vi "Main.vi"() -> ()   [LabVIEW 2020, in "Rename to match project.lvlib"]
uses:
  Rename to match project.lvlib
  process loops/Instrument Manager/Instrument State.ctl
  process loops/UI Manager/Data Display Loop Data.ctl
  process loops/Logging/Logging Configuration.ctl
  process loops/UI Manager/UI Data.ctl
  process loops/UI Manager/UI Display State.ctl
  Typedefs/System Control Data.ctl
  <vilib>/Utility/error.llb/Error Cluster From Error Code.vi
  <vilib>/ErrorRing/Error Ring.xnode
  support/Message Queue/Message Queue.lvlib
  support/User Event - Stop/User Event - Stop.lvlib
  process loops/Instrument Manager/Instrument Manager.lvlib
  process loops/Acquisition/Acquisition.lvlib
  process loops/Remote Connection Manager/Remote Connection Manager.lvlib
  process loops/Logging/Logging.lvlib
panel:
  in  "Time Interval (sec)":i32=1200
  out "Data Graph":cluster{timestamp[], dbl[]}[](graph)
  in  "Config Log Btn":bool
  in  "Sampling rate\n(sec/sample)":dbl=1.0 min=0.1 step=0.1
  in  "Log Data":bool
  in  "Stop Btn":bool=TRUE
  in  "Run Btn":bool
  out "Data Ind":dbl format="%d <u>"
  in  "Setpoint (units)":dbl format="%.3f"
  out "VISA resource":refnum<visa-resource-name>
  # "Plugin Template"
  # "Config"
  # "#CodeRecommended - To change display units, or remove them entirely, right click the display indicator >> Properties >> Display Format and replace or delete the <u>. If the rest of the format string is changed, be sure to change the Display Units cases in the UI Manager loop on the Block Diagram to reflect the changes."
  # "#CodePossibility - When plotting additional Instrument State data, right-click the Data Graph >> Properties >> Appearance and change the number of plots shown. Then go to the Plots tab and rename the plots to reflect the data being displayed."
  # "Instrument Control"
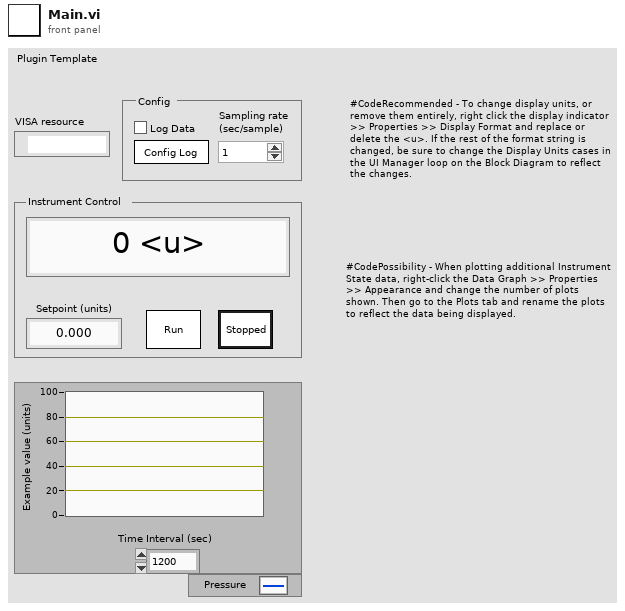
[diagram p1: front panel]
types:
  T1 = typedef "Rename to match project.lvlib/Data Display Loop Data.ctl" = cluster{"Data Timestamps":timestamp[], "Data Values":dbl[], "Previous Run State":bool}
  T2 = typedef "Rename to match project.lvlib/Instrument Manager.lvlib/Instrument State.ctl" = cluster{"VISA Resource":refnum<visa-resource-name>, "Setpoint":dbl, "Running":bool, "Running Since":timestamp, "Example Value Data Point":cluster{"Time Stamp":timestamp, "Value":dbl}, "Sampling Rate (sec/sample)":dbl}
  T3 = typedef "Rename to match project.lvlib/Message Queue.lvlib/All Message Queues.ctl" = cluster{"System Control":refnum<queue>, "Instrument":refnum<queue>, "Remote":refnum<queue>, "UI":refnum<queue>, "Acquisition":refnum<queue>, "Logging":refnum<queue>}
  T4 = typedef "Rename to match project.lvlib/UI Display State.ctl" = enum16{"Shown", "Hidden"}
  T5 = enum8{"Enabled", "Disabled", "Disabled and Grayed Out"}
  T6 = typedef "Rename to match project.lvlib/UI Data.ctl" = cluster{"VISA Resource Ind":refnum<vi>, "Setpoint Ctl":refnum<vi>, "Run Btn":refnum<vi>, "Stop Btn":refnum<vi>, "Data Ind":refnum<vi>, "Log Data":refnum<vi>, "Config Log Btn":refnum<vi>, "Sampling rate\n(sec/sample)":refnum<vi>, "Data Graph":refnum<vi>}
  T7 = typedef "Rename to match project.lvlib/Logging.lvlib/Logging Configuration.ctl" = cluster{"Log Directory Path":path, "Log File Path":path, "Log File Prefix":string, "Log File Extension":string, "File Delimiter":string, "Header Info":string[][], "Channels":string[], "Log Instrument Runs":bool}
  T8 = typedef "Rename to match project.lvlib/System Control Data.ctl" = cluster{"Example Value <Replace Me>":dbl, "Log Runs":bool, "Clone":bool}
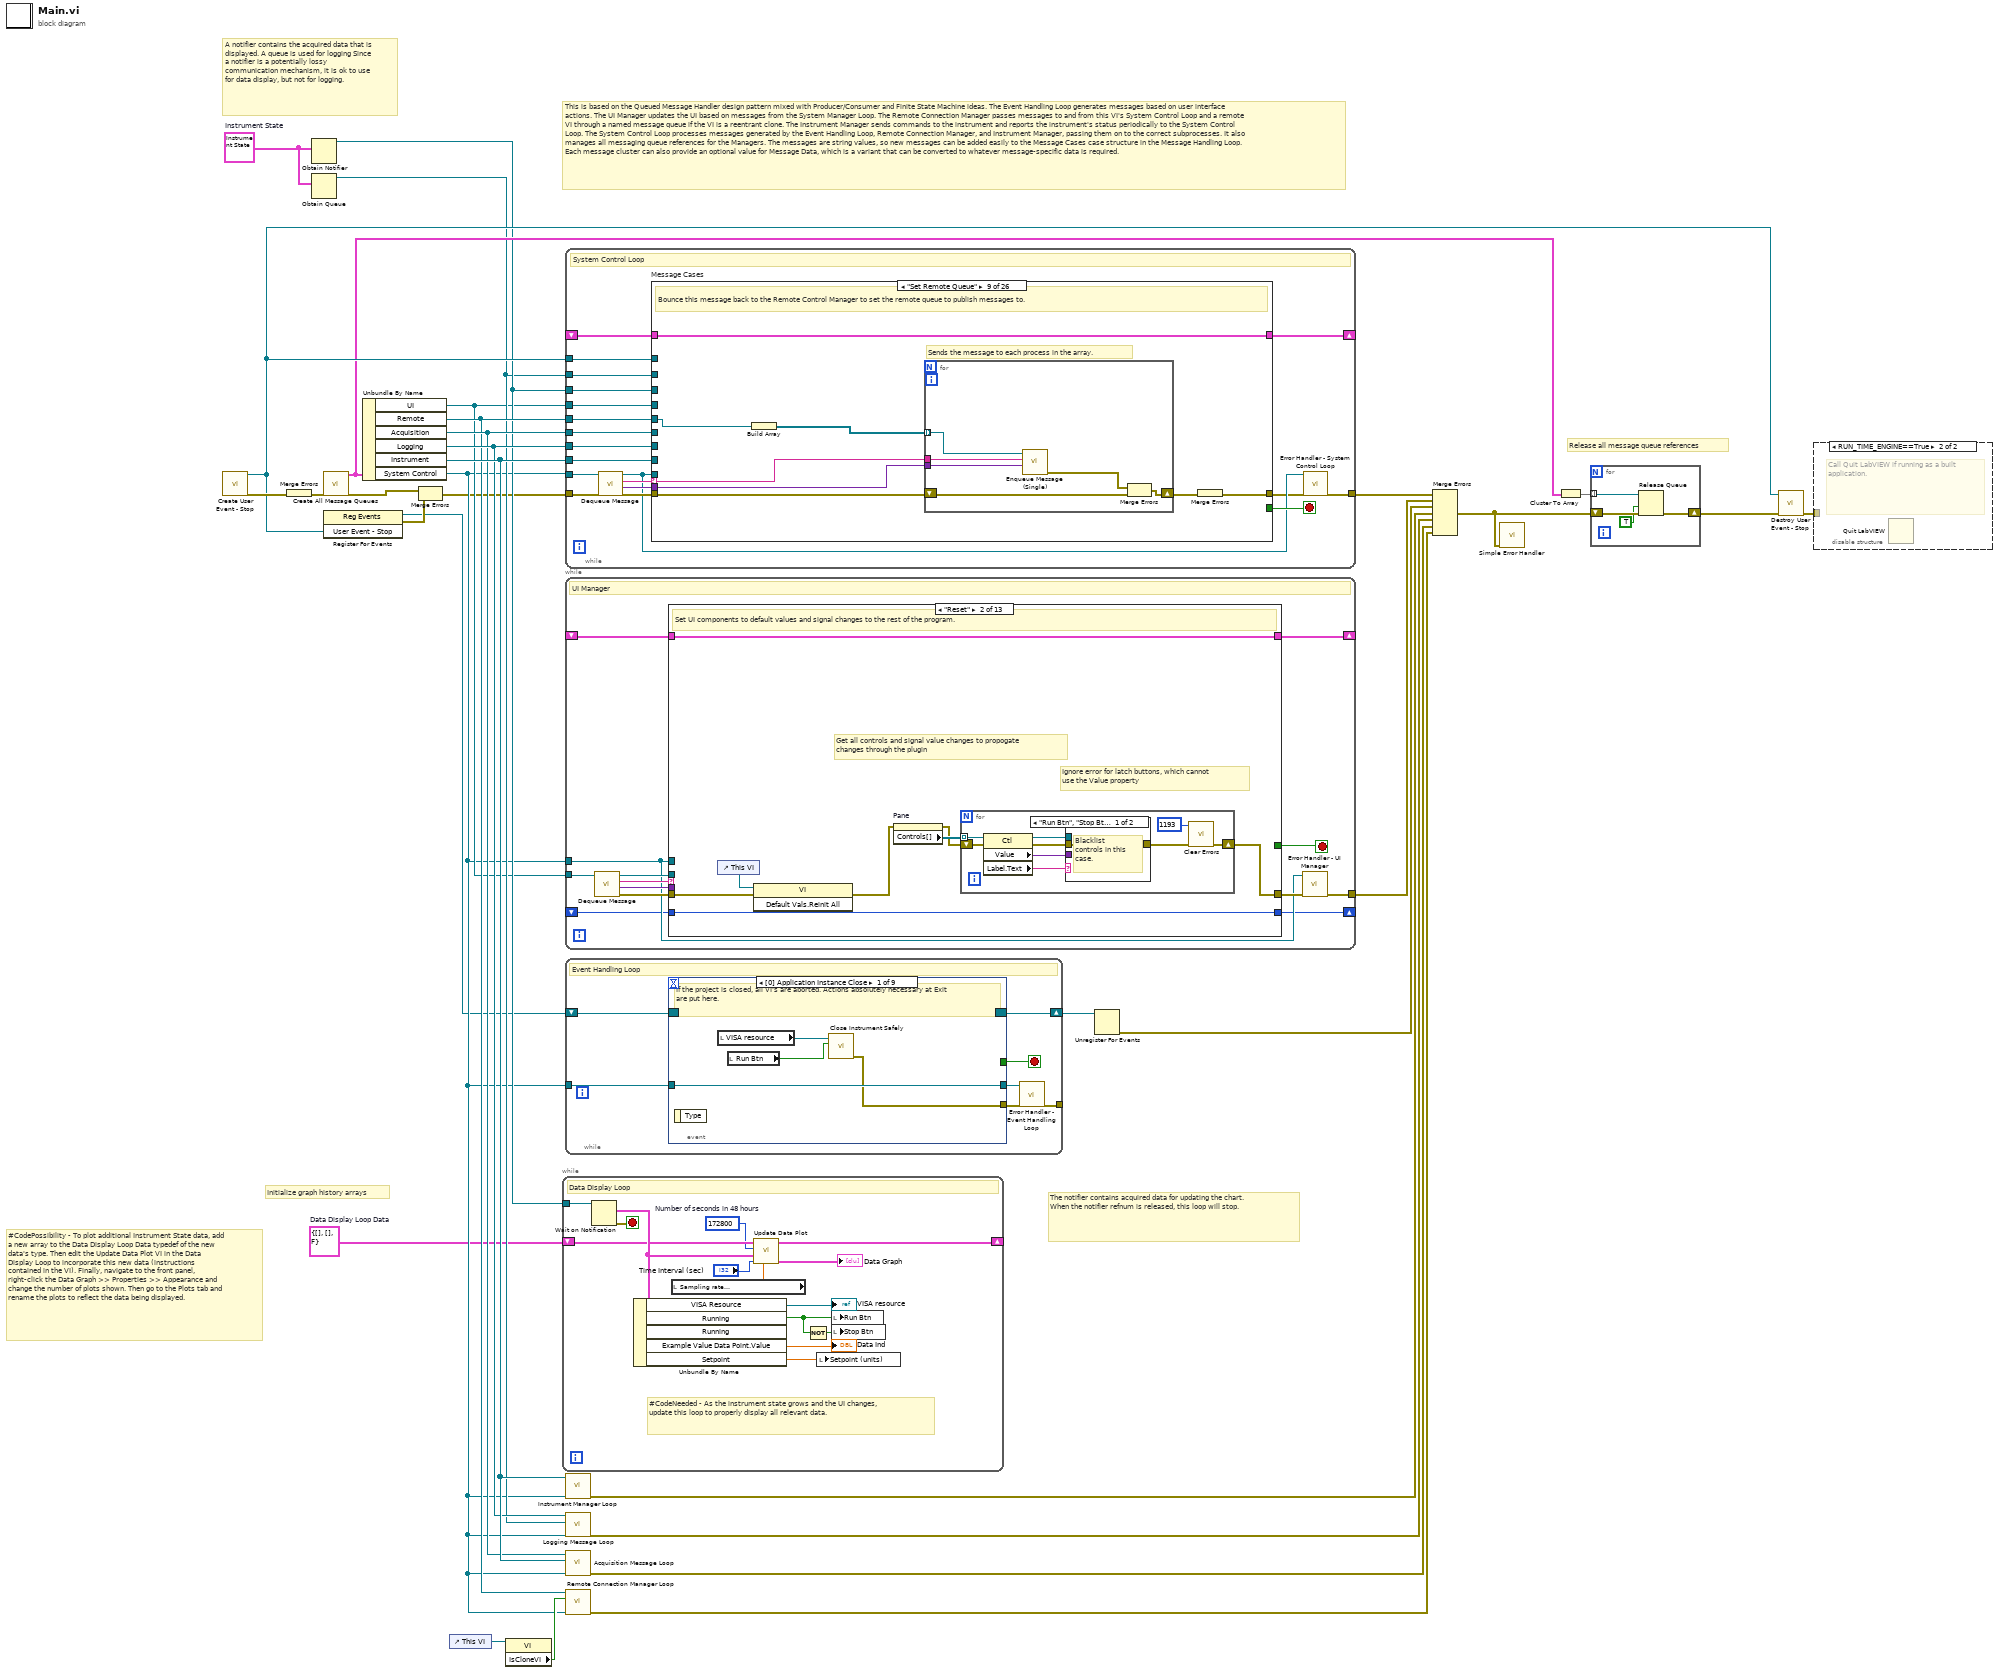
[diagram p0: block diagram]
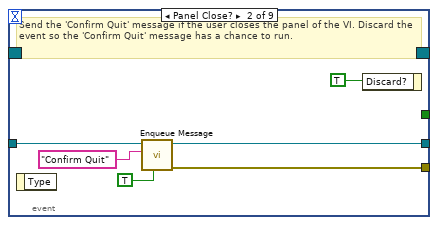
[diagram p2: hidden frame]
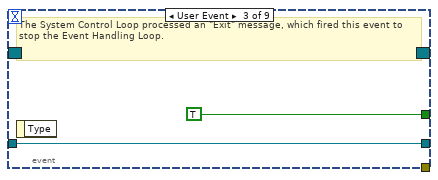
[diagram p3: hidden frame]
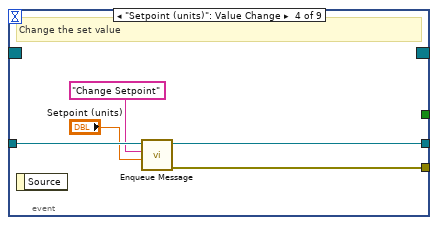
[diagram p4: hidden frame]
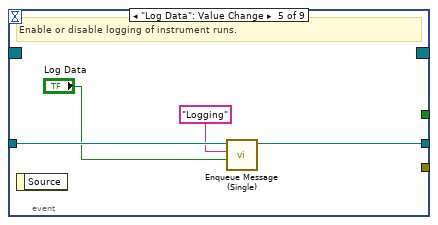
[diagram p5: hidden frame]
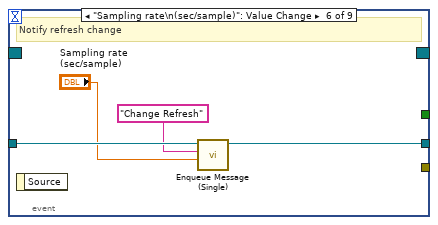
[diagram p6: hidden frame]
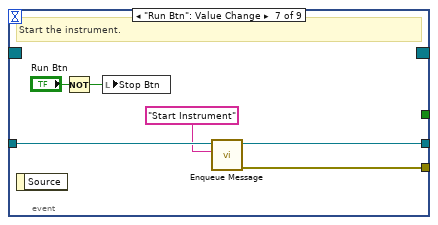
[diagram p7: hidden frame]
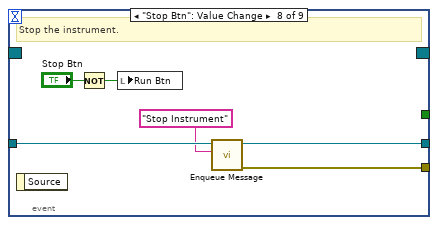
[diagram p8: hidden frame]
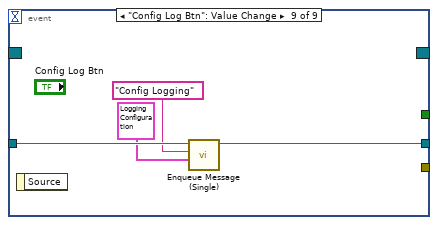
[diagram p9: hidden frame]
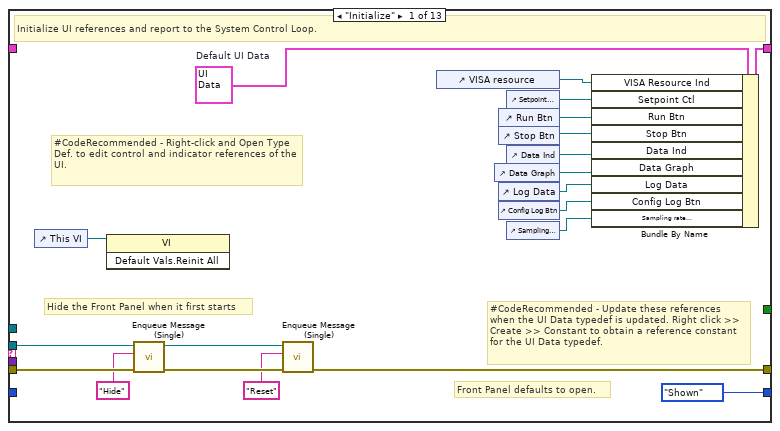
[diagram p10: hidden frame]
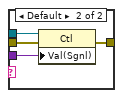
[diagram p11: hidden frame]
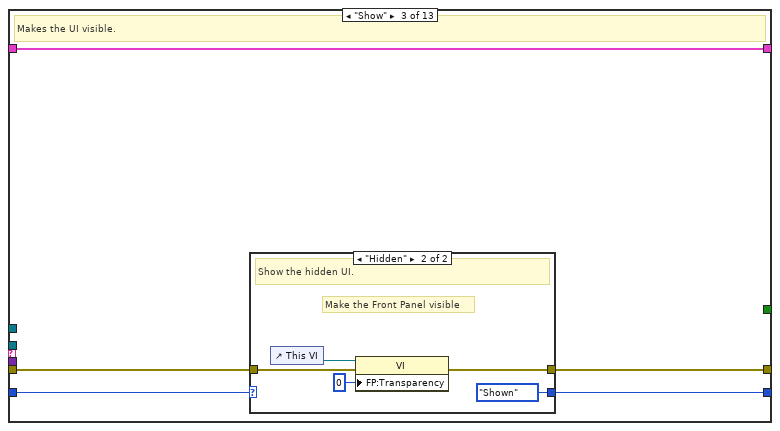
[diagram p12: hidden frame]
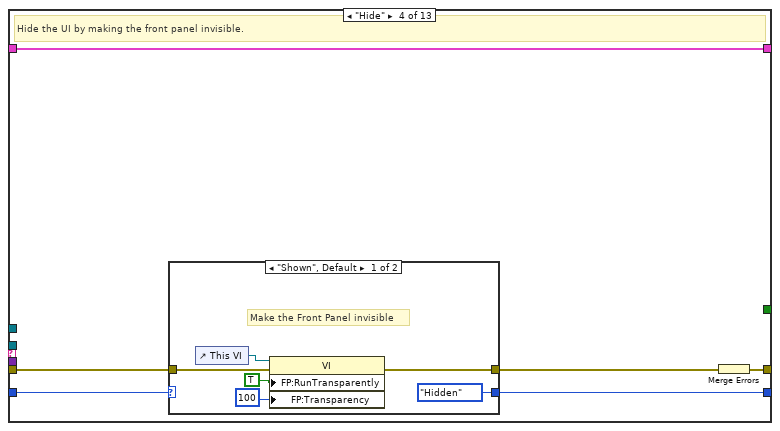
[diagram p14: hidden frame]
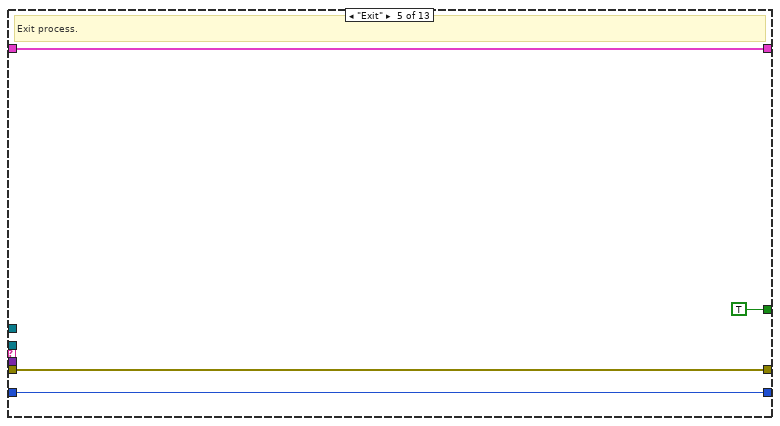
[diagram p16: hidden frame]
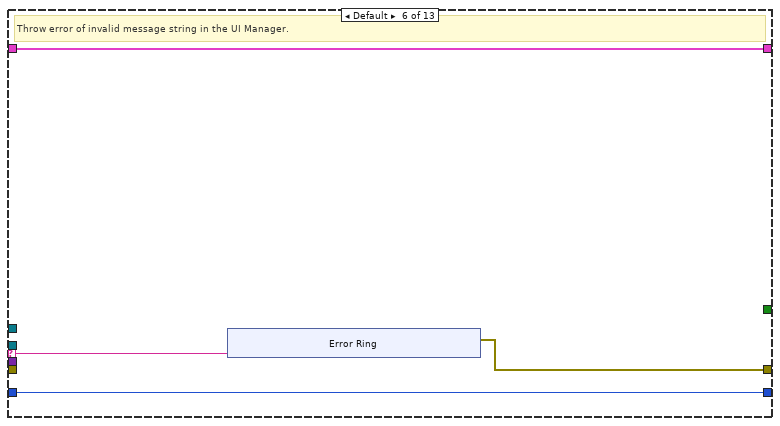
[diagram p17: hidden frame]
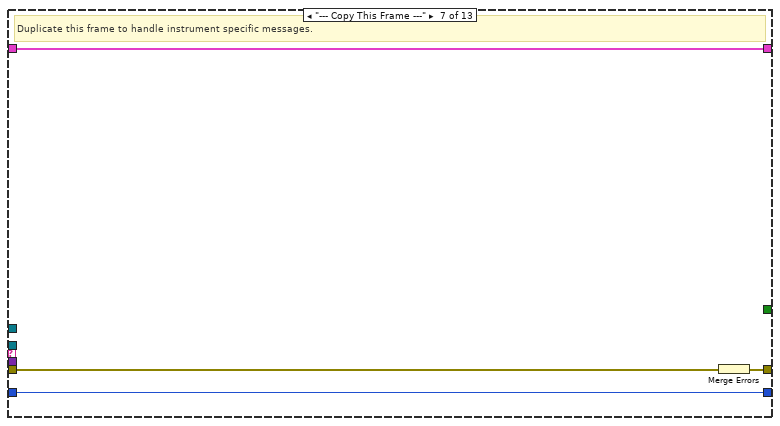
[diagram p18: hidden frame]
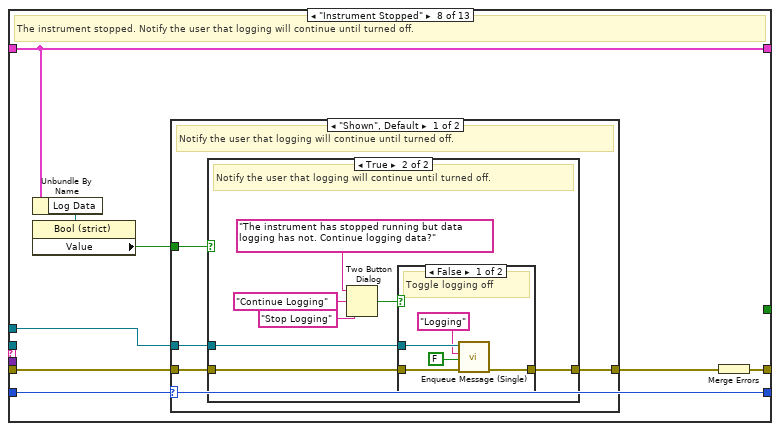
[diagram p19: hidden frame]
diagram:
  w1 = T1 {"Data Timestamps"=[], "Data Values"=[], "Previous Run State"=FALSE}  # Data Display Loop Data
  w7 = T2 {"VISA Resource"="", "Setpoint"=0.0, "Running"=FALSE, "Running Since"=timestamp(0 s since 1904-01-01), "Example Value Data Point"={"Time Stamp"=timestamp(0 s since 1904-01-01), "Value"=0.0}, "Sampling Rate (sec/sample)"=0.0}  # Instrument State
  # "#CodePossibility - To plot additional Instrument State data, add a new array to the Data Display Loop Data typedef of the new data's type. Then edit the Update Data Plot VI in the Data Display Loop to incorporate this new data (instructions contained in the VI). Finally, navigate to the front panel, right-click the Data Graph >> Properties >> Appearance and change the number of plots shown. Then go to the Plots tab and rename the plots to reflect the data being displayed."
  # "Initialize graph history arrays"
  # "A notifier contains the acquired data that is displayed. A queue is used for logging Since a notifier is a potentially lossy communication mechanism, it is ok to use for data display, but not for logging."
  # "The notifier contains acquired data for updating the chart. When the notifier refnum is released, this loop will stop."
  # "Release all message queue references"
  # "This is based on the Queued Message Handler design pattern mixed with Producer/Consumer and Finite State Machine ideas. The Event Handling Loop generates messages based on user interface actions. The UI Manager updates the UI based on messages from the System Manager Loop. The Remote Connection Manager passes messages to and from this VI's System Control Loop and a remote VI through a named message queue if the VI is a reentrant clone. The Instrument Manager sends commands to the instrument and reports the instrument's status periodically to the System Control Loop. The System Control Loop processes messages generated by the Event Handling Loop, Remote Connection Manager, and Instrument Manager, passing them on to the correct subprocesses. It also manages all messaging queue references for the Managers. The messages are string values, so new messages can be added easily to the Message Cases case structure in the Message Handling Loop.  Each message cluster can also provide an optional value for Message Data, which is a variant that can be converted to whatever message-specific data is required."
  n1 = call "Create User Event - Stop.vi"() -> ("error out"=w26:errorcluster, "User Event - Stop"=w22:refnum<user-event>)  [unwired: 10 in]
  n2 = Merge Errors(w26) -> (w25:errorcluster)
  n3 = Obtain Notifier(notification data type=w7) -> (notifier out=w8:refnum<notifier>)  [unwired: 3 in, 2 out]
  n4 = Obtain Queue(element data type=w7) -> (queue out=w6:refnum<queue>)  [unwired: 4 in, 2 out]
  n5 = call "Create All Message Queues.vi"("error in (no error)"=w25) -> ("error out"=w28:errorcluster, "Message Queues out"=w11:T3)  [unwired: 9 in]
  n6 = register-events(w22) -> (reference out=w2:refnum<event-registration>, error out=w13:errorcluster)  [unwired: 2 in]
  n7 = Unbundle By Name(w11) -> ("UI"=w5:refnum<queue>, "Remote"=w29:refnum<queue>, "Acquisition"=w30:refnum<queue>, "Logging"=w31:refnum<queue>, "Instrument"=w32:refnum<queue>, "System Control"=w4:refnum<queue>)
  n8 = Merge Errors(w28, w13) -> (w3:errorcluster)
  n9 = control-ref of="This VI"() -> (w21:refnum<vi>)
  n10 = property class="VI"(reference=w21) -> ("IsCloneVI"=w20:bool)  [unwired: 1 in, 2 out]
  n11 = while "Data Display Loop" {
    tunnel: w8 -> [w46]
    shift-right: [w36] -> _
    shift-left: w1 -> [w37]
    stop <- w45 stop-if-true
    w33 = 172800  # Number of seconds in 48 hours
    # "#CodeNeeded - As the instrument state grows and the UI changes, update this loop to properly display all relevant data."
    # "Data Display Loop"
    n12 = Wait on Notification(notifier=w46) -> (notification=w38:T2, error out=w45:errorcluster)  [unwired: 3 in, 2 out]
    n13 = Unbundle By Name(w38) -> ("VISA Resource"=→"VISA resource":refnum<visa-resource-name>, "Running"=w43:bool, "Example Value Data Point.Value"=→"Data Ind":dbl, "Setpoint"=w40:dbl)  [unwired: 1 out]
    n14 = local read "Sampling rate\n(sec/sample)"() -> (w34:dbl)
    n15 = call "Update Data Plot.vi"("Sample Rate (sec/sample)"=w34, "Time interval (s)"="Time Interval (sec)", "Instrument State"=w38, "History length (-1; unlimited)"=w33, "Graph History Arrays in"=w37) -> ("Updated Plot History"=→"Data Graph":cluster{timestamp[], dbl[]}[], "Graph History Arrays out"=w36:T1)  [unwired: 5 in]
    n16 = Not(x=w43) -> (.not. x?=w42:bool)
    n17 = local write "Setpoint (units)"(w40) -> ()
    n18 = local write "Run Btn"(w43) -> ()
    n19 = local write "Stop Btn"(w42) -> ()
  }
  n20 = while {
    tunnel: w5 -> [w59]
    tunnel: w4 -> [w50]
    tunnel: [w51] -> w19
    shift-right: [w54] -> _
    shift-left: _ -> [w53]
    shift-right: [w48] -> _
    shift-left: _ -> [w47]
    stop <- w49 stop-if-true
    # "UI Manager"
    n21 = call "Dequeue Message.vi"("Message Queue"=w59) -> ("error out"=w57:errorcluster, "Message Data"=w55:variant, "Message"=w56:string, "dup Message Queue"=w58:refnum<queue>)  [unwired: 7 in]
    n22 = case shown="\"Reset\"" w56 {
      selector: w56 -> [_ _ _ _ _ w135 _ _ _ _ _ _ _]
      tunnel: w58 -> [w71 _ _ _ _ _ _ _ _ _ _ _ _]
      tunnel: w57 -> [w76 w83 w105 w117 w131 _ w144 w152 w180 w188 w196 w211 w222]
      tunnel: w55 -> [_ _ _ _ _ _ _ _ _ _ w195 w209 w221]
      tunnel: w50 -> [_ _ _ _ _ _ _ w150 _ _ _ _ _]
      tunnel: [w62 w82 w104 w118 w131 w134 w145 w154 w181 w189 w197 w212 w223] -> w52
      tunnel: [w78 w80 w106 w119 w130 w133 w146 w149 w176 w182 w191 w204 w217] -> w54
      tunnel: w53 -> [_ w80 w106 w119 w130 w133 w146 w149 w176 w182 w191 w204 w217]
      tunnel: [_ _ _ _ TRUE _ _ _ _ _ _ _ _] -> w49
      tunnel: w47 -> [_ w81 w103 w115 w128 w132 w143 w153 w179 w187 w193 w205 w218]
      tunnel: [UI_Display_State."Shown" ("UI Display State") w81 w102 w114 w128 w132 w143 w153 w179 w187 w193 w205 w218] -> w48
      frame "Initialize" {
        w79 = T6 {"VISA Resource Ind"=refnum, "Setpoint Ctl"=refnum, "Run Btn"=refnum, "Stop Btn"=refnum, "Data Ind"=refnum, "Log Data"=refnum, "Config Log Btn"=refnum, "Sampling rate\n(sec/sample)"=refnum, "Data Graph"=refnum}  # Default UI Data
        # "Front Panel defaults to open."
        # "Hide the Front Panel when it first starts"
        # "#CodeRecommended - Update these references when the UI Data typedef is updated. Right click >> Create >> Constant to obtain a reference constant for the UI Data typedef."
        # "#CodeRecommended - Right-click and Open Type Def. to edit control and indicator references of the UI."
        # "Initialize UI references and report to the System Control Loop."
        n23 = control-ref of="This VI"() -> (w64:refnum<vi>)
        n24 = invoke class="VI" method="Default Vals.Reinit All"(reference=w64) -> ()  [unwired: 2 in, 3 out]
        n25 = call "Enqueue Message (Single).vi"("error in (no error)"=w76, "Message"="Hide", "Message Queue"=w71) -> ("error out"=w63:errorcluster, "dup Message Queue"=w61:refnum<queue>)  [unwired: 7 in]
        n26 = call "Enqueue Message (Single).vi"("error in (no error)"=w63, "Message"="Reset", "Message Queue"=w61) -> ("error out"=w62:errorcluster)  [unwired: 7 in, 1 out]
        n27 = control-ref of="VISA resource"() -> (w75:refnum<vi>)
        n28 = control-ref of="Data Graph"() -> (w68:refnum<vi>)
        n29 = control-ref of="Run Btn"() -> (w73:refnum<vi>)
        n30 = control-ref of="Stop Btn"() -> (w74:refnum<vi>)
        n31 = control-ref of="Log Data"() -> (w67:refnum<vi>)
        n32 = control-ref of="Config Log Btn"() -> (w66:refnum<vi>)
        n33 = control-ref of="Setpoint (units)"() -> (w77:refnum<vi>)
        n34 = control-ref of="Data Ind"() -> (w72:refnum<vi>)
        n35 = control-ref of="Sampling rate (sec/sample)"() -> (w65:refnum<vi>)
        n36 = Bundle By Name(cluster=w79, "VISA Resource Ind"=w75, "Setpoint Ctl"=w77, "Run Btn"=w73, "Stop Btn"=w74, "Data Ind"=w72, "Data Graph"=w68, "Log Data"=w67, "Config Log Btn"=w66, "Sampling rate\n(sec/sample)"=w65) -> (w78:T6)
      }
      frame "Reset" {
        # "Ignore error for latch buttons, which cannot\nuse the Value property"
        # "Get all controls and signal value changes to propogate\nchanges through the plugin"
        # "Set UI components to default values and signal changes to the rest of the program."
        n37 = control-ref of="This VI"() -> (w87:refnum<vi>)
        n38 = invoke class="VI" method="Default Vals.Reinit All"(reference=w87, error in=w83) -> (error out=w84:errorcluster)  [unwired: 1 in, 2 out]
        n39 = property on="Pane" class="Pane"(error in=w84) -> (error out=w85:errorcluster, "Controls[]"=w86:refnum<vi>[])  [unwired: 1 in, 1 out]
        n40 = for {
          tunnel: w86 -> [w96] mode=indexing
          shift-right: [w90] -> w82
          shift-left: w85 -> [w95]
          n41 = property class="Ctl"(reference=w96, error in=w95) -> (reference out=w94:refnum<vi>, error out=w93:errorcluster, "Value"=w92:variant, "Label.Text"=w88:string)
          n42 = case shown="\"Run Btn\", \"Stop Btn\"" w88 {
            tunnel: w94 -> [_ w101]
            tunnel: w93 -> [w97 w100]
            tunnel: w92 -> [_ w99]
            tunnel: [w97 w98] -> w91
            frame "Run Btn", "Stop Btn" {
              # "Blacklist controls in this case."
            }
            frame Default {
              n43 = property class="Ctl"(reference=w101, error in=w100, "Val(Sgnl)"=w99) -> (error out=w98:errorcluster)  [unwired: 1 out]
            }
          }
          n44 = call <vilib>:"Clear Errors.vi"("error in (no error)"=w91, "specific error code to clear (0: all)"=1193) -> ("error out"=w90:errorcluster)  [unwired: 4 in, 1 out]
        }
      }
      frame "Show" {
        # "Makes the UI visible."
        n45 = case shown="\"Hidden\"" w103 {
          selector: w103 -> [w108 _]
          tunnel: w105 -> [w107 w113]
          tunnel: [w107 w111] -> w104
          tunnel: [w108 UI_Display_State."Shown" ("UI Display State")] -> w102
          frame "Shown", Default {
            # "Do nothing if UI is already shown."
          }
          frame "Hidden" {
            # "Make the Front Panel visible"
            # "Show the hidden UI."
            n46 = control-ref of="This VI"() -> (w112:refnum<vi>)
            n47 = property class="VI"(reference=w112, error in=w113, "FP:Transparency"=u8 0 ("Front Panel Window:Transparency")) -> (error out=w111:errorcluster)  [unwired: 1 out]
          }
        }
      }
      frame "Hide" {
        # "Hide the UI by making the front panel invisible."
        n48 = case shown="\"Shown\", Default" w115 {
          selector: w115 -> [_ w127]
          tunnel: w117 -> [w122 w126]
          tunnel: [w121 w126] -> w116
          tunnel: [UI_Display_State."Hidden" ("UI Display State") w127] -> w114
          frame "Shown", Default {
            # "Make the Front Panel invisible"
            n49 = control-ref of="This VI"() -> (w125:refnum<vi>)
            n50 = property class="VI"(reference=w125, error in=w122, "FP:RunTransparently"=TRUE ("Front Panel Window:Run VI Transparently"), "FP:Transparency"=u8 100 ("Front Panel Window:Transparency")) -> (error out=w121:errorcluster)  [unwired: 1 out]
          }
          frame "Hidden" {
          }
        }
        n51 = Merge Errors(w116) -> (w118:errorcluster)
      }
      frame "Exit" {
        # "Exit process."
      }
      frame Default {
        # "Throw error of invalid message string in the UI Manager."
        n52 = xnode "Error Ring"("parameter 0"=w135) -> ("error out"=w134:errorcluster)
      }
      frame "--- Copy This Frame ---" {
        # "Duplicate this frame to handle instrument specific messages."
        n53 = Merge Errors(w144) -> (w145:errorcluster)
      }
      frame "Instrument Stopped" {
        # "The instrument stopped. Notify the user that logging will continue until turned off."
        n54 = Unbundle By Name(w149) -> ("Log Data"=w148:refnum<vi>)
        n55 = property class="Bool (strict)"(reference=w148) -> ("Value"=w147:bool)  [unwired: 1 in, 2 out]
        n56 = case shown="\"Shown\", Default" w153 {
          tunnel: w152 -> [w158 w173]
          tunnel: [w157 w173] -> w151
          tunnel: w150 -> [w156 _]
          tunnel: w147 -> [w155 _]
          frame "Shown", Default {
            # "Notify the user that logging will continue until turned off."
            n57 = case shown="True" w155 {
              tunnel: w158 -> [w159 w162]
              tunnel: [w159 w161] -> w157
              tunnel: w156 -> [_ w160]
              frame False {
                # "Not logging, do not show dialog"
              }
              frame True {
                # "Notify the user that logging will continue until turned off."
                n58 = Two Button Dialog(message="The instrument has stopped running but data logging has not. Continue logging data?", 1:"Stop Logging" ("F button name (\"Cancel\")"), 2:"Continue Logging" ("T button name (\"OK\")")) -> (T button?=w163:bool)
                n59 = case shown="False" w163 {
                  tunnel: w162 -> [w171 w172]
                  tunnel: [w170 w172] -> w161
                  tunnel: w160 -> [w169 _]
                  frame False {
                    # "Toggle logging off"
                    n60 = call "Enqueue Message (Single).vi"("error in (no error)"=w171, "Message Data"=FALSE, "Message"="Logging", "Message Queue"=w169) -> ("error out"=w170:errorcluster)  [unwired: 6 in, 1 out]
                  }
                  frame True {
                    # "Continues logging. Do nothing more"
                  }
                }
              }
            }
          }
          frame "Hidden" {
            # "Hidden, do not show dialog"
          }
        }
        n61 = Merge Errors(w151) -> (w154:errorcluster)
      }
      frame "Logging Started" {
        # "Indicate that logging started."
        n62 = Unbundle By Name(w176) -> ("Log Data"=w178:refnum<vi>)
        n63 = property class="Bool (strict)"(reference=w178, "Value"=TRUE ("Log Data")) -> ()  [unwired: 1 in, 2 out]
        n64 = Unbundle By Name(w176) -> ("Config Log Btn"=w175:refnum<vi>)
        n65 = property class="Bool"(reference=w175, "DisabledEnum"=T5."Disabled and Grayed Out" ("Disabled")) -> ()  [unwired: 1 in, 2 out]
        n66 = Merge Errors(w180) -> (w181:errorcluster)
      }
      frame "Logging Stopped" {
        # "Indicate that logging stopped."
        n67 = Unbundle By Name(w182) -> ("Log Data"=w186:refnum<vi>)
        n68 = property class="Bool (strict)"(reference=w186, "Value"=FALSE ("Log Data")) -> ()  [unwired: 1 in, 2 out]
        n69 = Unbundle By Name(w182) -> ("Config Log Btn"=w184:refnum<vi>)
        n70 = property class="Bool"(reference=w184, "DisabledEnum"=T5."Enabled" ("Disabled")) -> ()  [unwired: 1 in, 2 out]
        n71 = Merge Errors(w188) -> (w189:errorcluster)
      }
      frame "Change Refresh" {
        # "Update sample rate multiplier in the UI data chart and config indicator."
        n72 = Unbundle By Name(w191) -> ("Sampling rate\n(sec/sample)"=w192:refnum<vi>)
        n73 = Variant To Data(type=0.0, Variant=w195) -> (data=w190:dbl)  [unwired: 1 in, 1 out]
        n74 = property class="DigNum (strict)"(reference=w192, "Value"=w190) -> ()  [unwired: 1 in, 2 out]
        n75 = Merge Errors(w196) -> (w197:errorcluster)
      }
      frame "Update Example Value Units" {
        # "Change the units of the display."
        n76 = Variant To Data(type="", Variant=w209) -> (data=w199:string)  [unwired: 1 in, 1 out]
        n77 = call <vilib>:"Space Constant.vi"() -> ("String"=w208:string)
        n78 = Concatenate Strings("%d" ("string"), w208, w199) -> (w206:string)
        n79 = Unbundle By Name(w204) -> ("Data Ind"=w203:refnum<vi>, "Data Graph"=w198:refnum<vi>)
        n80 = Concatenate Strings("Example Value (" ("concatenated string"), w199, ")" ("string")) -> (w202:string)
        n81 = property on="Property Node" class="DigNum (strict)"(reference=w203, "FormatString"=w206) -> ()  [unwired: 1 in, 2 out]
        n82 = property class="XYGraph (strict)"(reference=w198, "YScale.NameLbl.Text"=w202) -> ()  [unwired: 1 in, 2 out]
        n83 = Merge Errors(w211) -> (w212:errorcluster)
      }
      frame "Update Setpoint Units" {
        # "Change the units of the setpoint display."
        n84 = Variant To Data(type="", Variant=w221) -> (data=w215:string)  [unwired: 1 in, 1 out]
        n85 = Concatenate Strings("Setpoint (" ("string"), w215, ")" ("string")) -> (w219:string)
        n86 = Unbundle By Name(w217) -> ("Setpoint Ctl"=w216:refnum<vi>)
        n87 = property on="Property Node" class="DigNum (strict)"(reference=w216, "FormatString"=w219) -> ()  [unwired: 1 in, 2 out]
        n88 = Merge Errors(w222) -> (w223:errorcluster)
      }
    }
    n89 = call "Error Handler - UI Manager.vi"("error in (no error)"=w52, "Message Queue"=w50) -> ("dup error in"=w51:errorcluster)  [unwired: 8 in, 1 out]
  }
  n90 = while {
    tunnel: w4 -> [w230]
    shift-right: [w228] -> w23
    shift-left: w2 -> [w229]
    tunnel: [w224] -> _
    stop <- w226 stop-if-true
    # "Event Handling Loop"
    n91 = event shown="[0] Application Instance Close" {
      selector: w229 -> [_ _ _ _ _ _ _ _ _]
      dyn-events: [_ _ _ _ _ _ _ _ _] -> w228
      timeout: _ -> [_ _ _ _ _ _ _ _ _]
      tunnel: [_ _ TRUE ("Discard?") _ _ _ _ _ _] -> w226
      tunnel: w230 -> [w234 w239 w242 w247 w251 w255 w261 w267 w271]
      tunnel: [w233 w238 _ w244 _ _ w259 w265 _] -> w227
      tunnel: [w234 w237 w242 w246 w250 w254 w260 w266 w270] -> w225
      event Application Instance Close {
        # "If the project is closed, all VI's are aborted. Actions absolutely necessary at Exit are put here."
        n92 = event-data() -> ()  [unwired: 1 in, 1 out]
        n93 = local read "VISA resource"() -> (w232:refnum<visa-resource-name>)
        n94 = local read "Run Btn"() -> (w231:bool)
        n95 = call "Close Instrument Safely.vi"("Running (F)"=w231, "VISA Refnum in"=w232) -> ("error out"=w233:errorcluster)  [unwired: 9 in]
      }
      event Panel Close? {
        # "Send the 'Confirm Quit' message if the user closes the panel of the VI. Discard the event so the 'Confirm Quit' message has a chance to run."
        n96 = event-data() -> ()  [unwired: 1 in, 1 out]
        n97 = call-poly "Enqueue Message.vi"("Priority Message? (F)"=TRUE, "Message"="Confirm Quit", "Message Queue"=w239) -> ("error out"=w238:errorcluster, "dup Message Queue"=w237:refnum<queue>)  [unwired: 7 in]
        n98 = event-data("Discard?"=TRUE) -> ()  [unwired: 1 in, 1 out]
      }
      event User Event {
        # "The System Control Loop processed an \"Exit\" message, which fired this event to stop the Event Handling Loop."
        n99 = event-data() -> ()  [unwired: 1 in, 1 out]
      }
      event "Setpoint (units)": Value Change {
        # "Change the set value"
        n100 = event-data() -> ()  [unwired: 1 in, 1 out]
        n101 = call-poly "Enqueue Message.vi"("Message Data"="Setpoint (units)", "Message"="Change Setpoint", "Message Queue"=w247) -> ("error out"=w244:errorcluster, "dup Message Queue"=w246:refnum<queue>)  [unwired: 7 in]
      }
      event "Log Data": Value Change {
        # "Enable or disable logging of instrument runs."
        n102 = event-data() -> ()  [unwired: 1 in, 1 out]
        n103 = call "Enqueue Message (Single).vi"("Message Data"="Log Data", "Message"="Logging", "Message Queue"=w251) -> ("dup Message Queue"=w250:refnum<queue>)  [unwired: 7 in, 1 out]
      }
      event "Sampling rate\n(sec/sample)": Value Change {
        # "Notify refresh change"
        n104 = event-data() -> ()  [unwired: 1 in, 1 out]
        n105 = call "Enqueue Message (Single).vi"("Message Data"="Sampling rate\n(sec/sample)", "Message"="Change Refresh", "Message Queue"=w255) -> ("dup Message Queue"=w254:refnum<queue>)  [unwired: 7 in, 1 out]
      }
      event "Run Btn": Value Change {
        # "Start the instrument."
        n106 = event-data() -> ()  [unwired: 1 in, 1 out]
        n107 = Not(x="Run Btn") -> (.not. x?=w256:bool)
        n108 = local write "Stop Btn"(w256) -> ()
        n109 = call-poly "Enqueue Message.vi"("Message"="Start Instrument", "Message Queue"=w261) -> ("error out"=w259:errorcluster, "dup Message Queue"=w260:refnum<queue>)  [unwired: 8 in]
      }
      event "Stop Btn": Value Change {
        # "Stop the instrument."
        n110 = event-data() -> ()  [unwired: 1 in, 1 out]
        n111 = Not(x="Stop Btn") -> (.not. x?=w262:bool)
        n112 = local write "Run Btn"(w262) -> ()
        n113 = call-poly "Enqueue Message.vi"("Message"="Stop Instrument", "Message Queue"=w267) -> ("error out"=w265:errorcluster, "dup Message Queue"=w266:refnum<queue>)  [unwired: 8 in]
      }
      event "Config Log Btn": Value Change {
        n114 = event-data() -> ()  [unwired: 1 in, 1 out]
        n115 = call "Enqueue Message (Single).vi"("Message Data"=T7 {"Log Directory Path"=path "", "Log File Path"=path "", "Log File Prefix"="Experiment", "Log File Extension"="csv", "File Delimiter"=",", "Header Info"=[], "Channels"=[], "Log Instrument Runs"=FALSE} ("Logging Configuration"), "Message"="Config Logging", "Message Queue"=w271) -> ("dup Message Queue"=w270:refnum<queue>)  [unwired: 7 in, 1 out]
      }
    }
    n116 = call "Error Handler - Event Handling Loop.vi"("error in (no error)"=w227, "Message Queue"=w225) -> ("dup error in"=w224:errorcluster)  [unwired: 8 in, 1 out]
  }
  n117 = call "Instrument Manager Loop.vi"("System Control"=w4, "Instrument Manager"=w32) -> ("error out"=w17:errorcluster)  [unwired: 9 in]
  n118 = call "Acquisition Message Loop.vi"("System Control"=w4, "Instrument Manager"=w32, "Acquisition"=w30) -> ("error out"=w15:errorcluster)  [unwired: 8 in]
  n119 = call "Remote Connection Manager Loop.vi"("System Control"=w4, "IsCloneVI (false)"=w20, "Remote"=w29) -> ("error out"=w14:errorcluster)  [unwired: 8 in]
  n120 = while {
    tunnel: w4 -> [w282]
    shift-right: [w289] -> _
    shift-left: _ -> [w290]
    tunnel: w22 -> [w287]
    tunnel: w3 -> [w286]
    tunnel: [w280] -> w27
    tunnel: w32 -> [w278]
    tunnel: w29 -> [w277]
    tunnel: w5 -> [w276]
    tunnel: w30 -> [w275]
    tunnel: w31 -> [w274]
    tunnel: w8 -> [w273]
    tunnel: w6 -> [w272]
    stop <- w288 stop-if-true
    # "System Control Loop"
    n121 = call "Dequeue Message.vi"("error in (no error)"=w286, "Message Queue"=w282) -> ("error out"=w285:errorcluster, "Message Data"=w283:variant, "Message"=w284:string, "dup Message Queue"=w281:refnum<queue>)  [unwired: 6 in]
    n122 = case "Message Cases" shown="\"Set Remote Queue\"" w284 {
      selector: w284 -> [_ _ _ w332 w345 w356 w376 w391 w404 w418 w424 _ w470 w477 w484 w491 w498 w508 w522 w537 w551 w562 w569 w579 w594 w616]
      tunnel: w281 -> [_ _ w312 _ _ _ _ _ _ _ _ _ _ _ _ _ _ _ _ _ _ _ _ _ _ _]
      tunnel: w285 -> [w294 w309 w316 _ _ w359 w379 w394 w407 w422 w440 w453 w474 w481 w488 w495 w502 w511 w525 w541 w555 w565 w572 _ _ _]
      tunnel: [w293 w303 w314 w335 w346 w365 w380 w395 w409 w423 w431 w458 w475 w482 w489 w496 w503 w512 w526 w539 w553 w566 w573 w578 w593 w615] -> w279
      tunnel: w290 -> [_ w308 w315 w331 w347 w366 w381 w396 w410 w421 w430 w459 w476 w483 w490 w497 w504 w513 w527 w540 w554 w567 w574 w577 w590 w613]
      tunnel: [w295 w308 w315 w331 w347 w366 w381 w396 w410 w421 w430 w457 w476 w483 w490 w497 w504 w513 w527 w540 w554 w567 w574 w577 w590 w613] -> w289
      tunnel: [_ _ _ TRUE _ _ _ _ _ _ _ _ _ _ _ _ _ _ _ _ _ _ _ _ _ _] -> w288
      tunnel: w283 -> [_ w307 _ w336 _ w355 w375 w390 w403 w417 w425 w455 w471 w478 w485 w492 w499 w509 w523 w536 w550 w563 w570 w580 w595 w611]
      tunnel: w287 -> [_ _ _ w333 _ _ _ _ _ _ _ _ _ _ _ _ _ _ _ _ _ _ _ _ _ _]
      tunnel: w278 -> [w292 _ _ w328 _ w360 _ _ _ w419 _ _ _ _ _ _ _ _ _ _ w549 w561 w568 _ _ _]
      tunnel: w277 -> [_ _ _ w327 _ w363 _ _ w408 _ w435 _ _ _ _ _ _ w507 w521 _ _ _ _ w581 w591 w614]
      tunnel: w276 -> [_ _ _ w326 _ w362 w373 w388 _ _ w434 _ _ _ _ _ _ w506 w520 w534 _ _ _ _ w589 _]
      tunnel: w275 -> [_ _ _ w330 _ w364 _ _ _ _ w437 _ _ _ _ _ _ _ _ w535 w548 _ _ w576 _ _]
      tunnel: w274 -> [_ _ _ w329 _ w361 w374 w389 _ _ w427 w451 w472 w479 w486 w493 w500 _ _ _ _ _ _ w575 _ _]
      tunnel: w273 -> [_ _ _ w323 _ _ _ _ _ _ _ _ _ _ _ _ _ _ _ _ _ _ _ _ _ w612]
      tunnel: w272 -> [_ _ _ w321 _ _ _ _ _ _ _ _ _ _ _ _ _ _ _ _ _ _ _ _ _ w608]
      frame "Initialize" {
        w296 = T8 {"Example Value <Replace Me>"=0.0, "Log Runs"=FALSE, "Clone"=FALSE}  # Default Data
        # "Initialize the system control loop and system."
        n123 = control-ref of="This VI"() -> ()  [unwired: 1 out]
        n124 = property on="Property Node" class="VI"() -> ("IsCloneVI"=w291:bool)  [unwired: 2 in, 2 out]
        n125 = Bundle By Name(cluster=w296, "Clone"=w291) -> (w295:T8)
        n126 = case shown="False" w291 {
          tunnel: w294 -> [w299 w302]
          tunnel: [w298 w302] -> w293
          tunnel: w292 -> [w297 _]
          frame False {
            # "Initiate the VISA Resource selection window if this is not a"
            n127 = call "Enqueue Message (Single).vi"("error in (no error)"=w299, "Message Data"=refnum<visa-resource-name> refnum ("VISA resource out"), "Message"="Set VISA Resource", "Message Queue"=w297) -> ("error out"=w298:errorcluster)  [unwired: 6 in, 1 out]
          }
          frame True {
            # "Reentrant clone. It is the responsibility of the RCM to send the Set VISA Resource command."
          }
        }
      }
      frame "Error" {
        # "#CodeRecommended - If you ever change the name of this \"Error\" message, you'll need to update the name in the Check Loop Error.vi as well."
        # "#CodeRecommended - Consider creating a system for logging errors in some way. These errors are for notification purposes only. Handling of specific errors should be performed in the message frames that generated the error."
        # "Error - Display an error dialog. This message is sent by the \"Error Handler\" VIs at the end of other loops in this application."
        n128 = Variant To Data(error in=w309, type=errorcluster {"status"=FALSE, "code"=0, "source"=""} ("error constant"), Variant=w307) -> (data=w305:errorcluster, error out=w304:errorcluster)
        n129 = call <vilib>:"Simple Error Handler.vi"("error in (no error)"=w305) -> ()  [unwired: 4 in, 5 out]
        n130 = Merge Errors(w304) -> (w303:errorcluster)
      }
      frame "Confirm Quit" {
        # "#CodeNeeded - If you want to provide an \"Are you sure\" dialog (or some other notification) before the application exits, place that code here. This message is typically sent from a Panel Close? event."
        # "Confirm Quit - Message that can confirm whether or not the user wants to exit the application."
        n131 = call-poly "Enqueue Message.vi"("Priority Message? (F)"=TRUE, "error in (no error)"=w316, "Message"="Exit", "Message Queue"=w312) -> ("error out"=w313:errorcluster)  [unwired: 6 in, 1 out]
        n132 = Merge Errors(w313) -> (w314:errorcluster)
      }
      frame "Exit" {
        # "Order other processes to exit"
        # "Begin the application closing procedure by sending \"Exit\" commands to all running processes."
        n133 = Variant To Data(type=errorcluster {"status"=FALSE, "code"=0, "source"=""} ("error constant"), Variant=w336) -> (data=w337:errorcluster)  [unwired: 1 in, 1 out]
        n134 = Build Array(w326, w327, w330, w329, w328) -> (w325:refnum<queue>[])
        n135 = call <vilib>:"Clear Errors.vi"("error in (no error)"=w337, "specific error code to clear (0: all)"=5000) -> ("error out"=w318:errorcluster)  [unwired: 4 in, 1 out]
        n136 = call <vilib>:"Simple Error Handler.vi"("error in (no error)"=w318) -> ()  [unwired: 4 in, 5 out]
        n137 = for {
          tunnel: w332 -> [w343]
          tunnel: w325 -> [w342] mode=indexing
          shift-right: [w341] -> w334
          shift-left: _ -> [w340]
          n138 = call "Enqueue Message (Single).vi"("Priority Message? (F)"=TRUE, "Message"=w343, "Message Queue"=w342) -> ("error out"=w344:errorcluster)  [unwired: 7 in, 1 out]
          n139 = Merge Errors(w344, w340) -> (w341:errorcluster)
        }
        n140 = Release Notifier(notifier=w323) -> (error out=w322:errorcluster)  [unwired: 2 in, 2 out]
        n141 = Release Queue(queue=w321) -> (error out=w319:errorcluster)  [unwired: 2 in, 2 out]
        n142 = call "Fire User Event - Stop.vi"("User Event - Stop"=w333) -> ("error out"=w320:errorcluster)  [unwired: 10 in]
        n143 = Merge Errors(w320, w319, w322, w334) -> (w335:errorcluster)
      }
      frame Default {
        # "'Default' case only runs if there is a message that isn't defined in any of the other cases.  Output a programming error."
        n144 = xnode "Error Ring"("parameter 0"=w345) -> ("error out"=w346:errorcluster)
      }
      frame "---Copy This Frame---" {
        # "Sends the message to each process in the array."
        # "#CodeRecommended - Change connections to build an array of the processes that will receive this message"
        # "Duplicate this frame when creating new messages.  Change this comment in the duplicated frame to describe this message."
        n145 = Build Array(w362, w363, w364, w361, w360) -> (w357:refnum<queue>[])
        n146 = for {
          tunnel: w357 -> [w370] mode=indexing
          tunnel: w356 -> [w372]
          tunnel: w355 -> [w371]
          shift-right: [w369] -> w358
          shift-left: w359 -> [w367]
          n147 = call "Enqueue Message (Single).vi"("Message Data"=w371, "Message"=w372, "Message Queue"=w370) -> ("error out"=w368:errorcluster)  [unwired: 7 in, 1 out]
          n148 = Merge Errors(w368, w367) -> (w369:errorcluster)
        }
        n149 = Merge Errors(w358) -> (w365:errorcluster)
      }
      frame "Update Example Value Units" {
        # "Sends the message to each process in the array."
        # "Change the Example Value units."
        n150 = Build Array(w373, w374) -> (w377:refnum<queue>[])
        n151 = for {
          tunnel: w377 -> [w385] mode=indexing
          tunnel: w376 -> [w387]
          tunnel: w375 -> [w386]
          shift-right: [w384] -> w378
          shift-left: w379 -> [w382]
          n152 = call "Enqueue Message (Single).vi"("Message Data"=w386, "Message"=w387, "Message Queue"=w385) -> ("error out"=w383:errorcluster)  [unwired: 7 in, 1 out]
          n153 = Merge Errors(w383, w382) -> (w384:errorcluster)
        }
        n154 = Merge Errors(w378) -> (w380:errorcluster)
      }
      frame "Update Setpoint Units" {
        # "Sends the message to each process in the array."
        # "Change the flow rate units."
        n155 = Build Array(w388, w389) -> (w392:refnum<queue>[])
        n156 = for {
          tunnel: w392 -> [w400] mode=indexing
          tunnel: w391 -> [w402]
          tunnel: w390 -> [w401]
          shift-right: [w399] -> w393
          shift-left: w394 -> [w397]
          n157 = call "Enqueue Message (Single).vi"("Message Data"=w401, "Message"=w402, "Message Queue"=w400) -> ("error out"=w398:errorcluster)  [unwired: 7 in, 1 out]
          n158 = Merge Errors(w398, w397) -> (w399:errorcluster)
        }
        n159 = Merge Errors(w393) -> (w395:errorcluster)
      }
      frame "Set Remote Queue" {
        # "Sends the message to each process in the array."
        # "Bounce this message back to the Remote Control Manager to set the remote queue to publish messages to."
        n160 = Build Array(w408) -> (w405:refnum<queue>[])
        n161 = for {
          tunnel: w405 -> [w414] mode=indexing
          tunnel: w404 -> [w416]
          tunnel: w403 -> [w415]
          shift-right: [w413] -> w406
          shift-left: w407 -> [w411]
          n162 = call "Enqueue Message (Single).vi"("Message Data"=w415, "Message"=w416, "Message Queue"=w414) -> ("error out"=w412:errorcluster)  [unwired: 7 in, 1 out]
          n163 = Merge Errors(w412, w411) -> (w413:errorcluster)
        }
        n164 = Merge Errors(w406) -> (w409:errorcluster)
      }
      frame "Set VISA Resource" {
        # "Update the VISA Resource of the instrument."
        n165 = call "Enqueue Message (Single).vi"("error in (no error)"=w422, "Message Data"=w417, "Message"=w418, "Message Queue"=w419) -> ("error out"=w420:errorcluster)  [unwired: 6 in, 1 out]
        n166 = Merge Errors(w420) -> (w423:errorcluster)
      }
      frame "Valid VISA Resource" {
        # "When a Valid VISA Resource has been chosen, start the other processes."
        n167 = Unbundle By Name(w430) -> ("Log Runs"=w429:bool)
        n168 = call "Enqueue Message (Single).vi"("error in (no error)"=w440, "Message Data"=w425, "Message"=w424, "Message Queue"=w427) -> ("error out"=w428:errorcluster, "dup Message Queue"=w426:refnum<queue>)  [unwired: 6 in]
        n169 = case shown="True" w429 {
          tunnel: w428 -> [w441 w445]
          tunnel: w426 -> [_ w444]
          tunnel: [w441 w442] -> w438
          frame False {
          }
          frame True {
            n170 = call "Enqueue Message (Single).vi"("error in (no error)"=w445, "Message"="Start", "Message Queue"=w444) -> ("error out"=w442:errorcluster)  [unwired: 7 in, 1 out]
          }
        }
        n171 = call "Enqueue Message (Single).vi"("error in (no error)"=w438, "Message"="Start", "Message Queue"=w437) -> ("error out"=w436:errorcluster)  [unwired: 7 in, 1 out]
        n172 = Unbundle By Name(w430) -> ("Clone"=w432:bool)
        n173 = call "Enqueue Message (Single).vi"("error in (no error)"=w436, "Message Data"=w425, "Message"=w424, "Message Queue"=w435) -> ("error out"=w433:errorcluster)  [unwired: 6 in, 1 out]
        n174 = case shown="False" w432 {
          tunnel: w433 -> [w449 w450]
          tunnel: [w448 w450] -> w431
          tunnel: w434 -> [w447 _]
          frame False {
            # "Show the Front Panel automatically on startup"
            n175 = call "Enqueue Message (Single).vi"("error in (no error)"=w449, "Message"="Show", "Message Queue"=w447) -> ("error out"=w448:errorcluster)  [unwired: 7 in, 1 out]
          }
          frame True {
            # "Reentrant clone. It is the responsibility of the RCM to send \"Show\"."
          }
        }
      }
      frame "Logging" {
        # "Enable or disable logging in the System Data. Run logging is disabled by default."
        n176 = Variant To Data(type=TRUE, Variant=w455) -> (data=w454:bool)  [unwired: 1 in, 1 out]
        n177 = case shown="True" w454 {
          tunnel: w453 -> [w464 w469]
          tunnel: [w463 w468] -> w452
          tunnel: w451 -> [w462 w467]
          frame False {
            n178 = call "Enqueue Message (Single).vi"("Priority Message? (F)"=TRUE, "error in (no error)"=w464, "Message"="Stop", "Message Queue"=w462) -> ("error out"=w463:errorcluster)  [unwired: 6 in, 1 out]
          }
          frame True {
            n179 = call "Enqueue Message (Single).vi"("Priority Message? (F)"=TRUE, "error in (no error)"=w469, "Message"="Start", "Message Queue"=w467) -> ("error out"=w468:errorcluster)  [unwired: 6 in, 1 out]
          }
        }
        n180 = Bundle By Name(cluster=w459, "Log Runs"=w454) -> (w457:T8)
        n181 = Merge Errors(w452) -> (w458:errorcluster)
      }
      frame "Config Logging" {
        # "Pass on Config Logging message to Logging Loop."
        n182 = call "Enqueue Message (Single).vi"("error in (no error)"=w474, "Message Data"=w471, "Message"=w470, "Message Queue"=w472) -> ("error out"=w473:errorcluster)  [unwired: 6 in, 1 out]
        n183 = Merge Errors(w473) -> (w475:errorcluster)
      }
      frame "Set Log Directory" {
        # "Pass on log setting message to Logging Loop."
        n184 = call "Enqueue Message (Single).vi"("error in (no error)"=w481, "Message Data"=w478, "Message"=w477, "Message Queue"=w479) -> ("error out"=w480:errorcluster)  [unwired: 6 in, 1 out]
        n185 = Merge Errors(w480) -> (w482:errorcluster)
      }
      frame "Set Log File Prefix" {
        # "Pass on log setting message to Logging Loop."
        n186 = call "Enqueue Message (Single).vi"("error in (no error)"=w488, "Message Data"=w485, "Message"=w484, "Message Queue"=w486) -> ("error out"=w487:errorcluster)  [unwired: 6 in, 1 out]
        n187 = Merge Errors(w487) -> (w489:errorcluster)
      }
      frame "Set Log File Delimiter" {
        # "Pass on log setting message to Logging Loop."
        n188 = call "Enqueue Message (Single).vi"("error in (no error)"=w495, "Message Data"=w492, "Message"=w491, "Message Queue"=w493) -> ("error out"=w494:errorcluster)  [unwired: 6 in, 1 out]
        n189 = Merge Errors(w494) -> (w496:errorcluster)
      }
      frame "Set Log on Run" {
        # "Pass on log setting message to Logging Loop."
        n190 = call "Enqueue Message (Single).vi"("error in (no error)"=w502, "Message Data"=w499, "Message"=w498, "Message Queue"=w500) -> ("error out"=w501:errorcluster)  [unwired: 6 in, 1 out]
        n191 = Merge Errors(w501) -> (w503:errorcluster)
      }
      frame "Logging Started" {
        # "Pass on Logging Started message to RCM and UI."
        n192 = Build Array(w506, w507) -> (w505:refnum<queue>[])
        n193 = for {
          tunnel: w509 -> [w516]
          tunnel: w508 -> [w515]
          shift-right: [w517] -> w510
          shift-left: w511 -> [w518]
          tunnel: w505 -> [w514] mode=indexing
          n194 = call "Enqueue Message (Single).vi"("error in (no error)"=w518, "Message Data"=w516, "Message"=w515, "Message Queue"=w514) -> ("error out"=w517:errorcluster)  [unwired: 6 in, 1 out]
        }
        n195 = Merge Errors(w510) -> (w512:errorcluster)
      }
      frame "Logging Stopped" {
        # "Pass on Logging Stopped message to RCM and UI."
        n196 = Build Array(w520, w521) -> (w519:refnum<queue>[])
        n197 = for {
          tunnel: w523 -> [w530]
          tunnel: w522 -> [w529]
          shift-right: [w531] -> w524
          shift-left: w525 -> [w532]
          tunnel: w519 -> [w528] mode=indexing
          n198 = call "Enqueue Message (Single).vi"("error in (no error)"=w532, "Message Data"=w530, "Message"=w529, "Message Queue"=w528) -> ("error out"=w531:errorcluster)  [unwired: 6 in, 1 out]
        }
        n199 = Merge Errors(w524) -> (w526:errorcluster)
      }
      frame "Change Refresh" {
        # "#CodePossibility - The default refresh rate can be changed by changing the default value of the front panel control."
        # "Change the sampling rate of the instrument. Default value is the default set on the front panel control."
        n200 = Build Array(w534, w535) -> (w533:refnum<queue>[])
        n201 = for {
          tunnel: w537 -> [w544]
          tunnel: w536 -> [w543]
          tunnel: w533 -> [w542] mode=indexing
          shift-right: [w545] -> w538
          shift-left: w541 -> [w546]
          n202 = call "Enqueue Message (Single).vi"("error in (no error)"=w546, "Message Data"=w543, "Message"=w544, "Message Queue"=w542) -> ("error out"=w545:errorcluster)  [unwired: 6 in, 1 out]
        }
        n203 = Merge Errors(w538) -> (w539:errorcluster)
      }
      frame "Change Setpoint" {
        # "Forward the Change Setpoint command to the IML and acquisition."
        n204 = Build Array(w548, w549) -> (w547:refnum<queue>[])
        n205 = for {
          tunnel: w551 -> [w558]
          tunnel: w550 -> [w557]
          shift-right: [w559] -> w552
          shift-left: w555 -> [w560]
          tunnel: w547 -> [w556] mode=indexing
          n206 = call "Enqueue Message (Single).vi"("error in (no error)"=w560, "Message Data"=w557, "Message"=w558, "Message Queue"=w556) -> ("error out"=w559:errorcluster)  [unwired: 6 in, 1 out]
        }
        n207 = Merge Errors(w552) -> (w553:errorcluster)
      }
      frame "Start Instrument" {
        # "Pass message to Instrument Manager Loop."
        n208 = call "Enqueue Message (Single).vi"("error in (no error)"=w565, "Message Data"=w563, "Message"=w562, "Message Queue"=w561) -> ("error out"=w564:errorcluster)  [unwired: 6 in, 1 out]
        n209 = Merge Errors(w564) -> (w566:errorcluster)
      }
      frame "Stop Instrument" {
        # "Pass message to Instrument Manager Loop."
        n210 = call "Enqueue Message (Single).vi"("error in (no error)"=w572, "Message Data"=w570, "Message"=w569, "Message Queue"=w568) -> ("error out"=w571:errorcluster)  [unwired: 6 in, 1 out]
        n211 = Merge Errors(w571) -> (w573:errorcluster)
      }
      frame "Instrument Started" {
        # "Build an array of all processes that will receive this message"
        # "Notify processes of update"
        # "Notify processes that the instrument is running."
        n212 = Build Array(w581, w576, w575) -> (w582:refnum<queue>[])
        n213 = for {
          tunnel: w582 -> [w586] mode=indexing
          tunnel: w579 -> [w588]
          tunnel: w580 -> [w587]
          shift-right: [w585] -> w578
          shift-left: _ -> [w583]
          n214 = call "Enqueue Message (Single).vi"("Message Data"=w587, "Message"=w588, "Message Queue"=w586) -> ("error out"=w584:errorcluster)  [unwired: 7 in, 1 out]
          n215 = Merge Errors(w584, w583) -> (w585:errorcluster)
        }
      }
      frame "Instrument Stopped" {
        # "Build an array of all processes that will receive this message"
        # "Notify processes of update"
        # "Notify processes that the instrument stopped running."
        n216 = Build Array(w589, w591) -> (w592:refnum<queue>[])
        n217 = for {
          tunnel: w592 -> [w599] mode=indexing
          tunnel: w594 -> [w601]
          tunnel: w595 -> [w600]
          shift-right: [w598] -> w593
          shift-left: _ -> [w596]
          n218 = call "Enqueue Message (Single).vi"("Message Data"=w600, "Message"=w601, "Message Queue"=w599) -> ("error out"=w597:errorcluster)  [unwired: 7 in, 1 out]
          n219 = Merge Errors(w597, w596) -> (w598:errorcluster)
        }
      }
      frame "Report" {
        # "Send instrument state notification"
        # "Notify processes that the instrument stopped running."
        n220 = Variant To Data(type=T2 {"VISA Resource"="", "Setpoint"=0.0, "Running"=FALSE, "Running Since"=timestamp(0 s since 1904-01-01), "Example Value Data Point"={"Time Stamp"=timestamp(0 s since 1904-01-01), "Value"=0.0}, "Sampling Rate (sec/sample)"=0.0} ("Instrument State"), Variant=w611) -> (data=w607:T2)  [unwired: 1 in, 1 out]
        n221 = local read "Sampling rate\n(sec/sample)"() -> (w603:dbl)
        n222 = Bundle By Name(cluster=w607, "Sampling Rate (sec/sample)"=w603) -> (w602:T2)
        n223 = Enqueue Element(queue=w608, element=w602) -> (error out=w605:errorcluster)  [unwired: 2 in, 2 out]
        n224 = Send Notification(notification=w602, notifier=w612) -> (error out=w609:errorcluster)  [unwired: 1 in, 1 out]
        n225 = Merge Errors(w605, w609) -> (w606:errorcluster)
        n226 = call "Enqueue Message (Single).vi"("Message Data"=w602, "Message"=w616, "Message Queue"=w614) -> ("error out"=w604:errorcluster)  [unwired: 7 in, 1 out]
        n227 = Merge Errors(w604, w606) -> (w615:errorcluster)
      }
    }
    n228 = call "Error Handler - System Control Loop.vi"("error in (no error)"=w279, "Message Queue"=w281) -> ("dup error in"=w280:errorcluster)  [unwired: 8 in, 1 out]
  }
  n229 = call "Logging Message Loop.vi"("System Control"=w4, "Data Queue"=w6, "Logging"=w31) -> ("error out"=w16:errorcluster)  [unwired: 8 in]
  n230 = Unregister For Events(event registration refnum=w23) -> (error out=w18:errorcluster)  [unwired: 1 in]
  n231 = Merge Errors(w27, w19, w18, w17, w16, w15, w14) -> (w12:errorcluster)
  n232 = call <vilib>:"Simple Error Handler.vi"("error in (no error)"=w12) -> ()  [unwired: 4 in, 5 out]
  n233 = Cluster To Array(cluster=w11) -> (array=w10:refnum<queue>[])
  n234 = for {
    shift-right: [w618] -> w9
    shift-left: w12 -> [w619]
    tunnel: w10 -> [w620] mode=indexing
    n235 = Release Queue(queue=w620, force destroy? (F)=TRUE, error in (no error)=w619) -> (error out=w618:errorcluster)  [unwired: 2 out]
  }
  n236 = call "Destroy User Event - Stop.vi"("error in (no error)"=w9, "User Event - Stop"=w22) -> ("error out"=w24:errorcluster)  [unwired: 9 in]
  n237 = disable-structure shown="RUN_TIME_ENGINE==True" {
    disable-tunnel: w24 -> [_ _]
    frame condition #0 (active) {
    }
    frame condition #1 {
      # "Call Quit LabVIEW if running as a built application."
      n238 = Quit LabVIEW() -> ()  [unwired: 1 in]
    }
  }
